vi "Drive_Globals.vi"() -> ()   [LabVIEW 2019]
uses:
  Subsystems/Drive/Drive_Cluster.ctl
  Subsystems/Drive/Drive_States.ctl
panel:
  in  "Swerve_IMU":string="Swerve_IMU"
  in  "Swerve_Drive_Front_Right_Ref":string="Swerve_Drive_Front_Right_Ref"
  in  "Swerve_Azimuth_Front_Right_Ref":string="Swerve_Azimuth_Front_Right_Ref"
  in  "Swerve_Drive_Back_Right_Ref":string="Swerve_Drive_Back_Right_Ref"
  in  "Swerve_Azimuth_Back_Right_Ref":string="Swerve_Azimuth_Back_Right_Ref"
  in  "Swerve_Drive_Back_Left_Ref":string="Swerve_Drive_Back_Left_Ref"
  in  "Swerve_Azimuth_Back_Left_Ref":string="Swerve_Azimuth_Back_Left_Ref"
  in  "Swerve_Drive_Front_Left_Ref":string="Swerve_Drive_Front_Left_Ref"
  in  "Swerve_Azimuth_Front_Left_Ref":string="Swerve_Azimuth_Front_Left_Ref"
  in  "Azimuth_Motor_Back_Right":dbl
  in  "Azimuth_Motor_Back_Left":dbl
  in  "Azimuth_Motor_Front_Left":dbl
  in  "Azimuth_Motor_Front_Right":dbl
  in  "Drive_Motor_Back_Right":dbl
  in  "Drive_Motor_Back_Left":dbl
  in  "Drive_Motor_Front_Left":dbl
  in  "Drive_Motor_Front_Right":dbl
  in  "Drive_Execute_Ref":string="Drive_Execute_Ref"
  in  "Drive_Set_Ref":string="Drive_Set_Ref"
  in  "Drive_Execute_Notifier":refnum<notifier>
  in  "Drive_Set_Notifier":refnum<notifier>
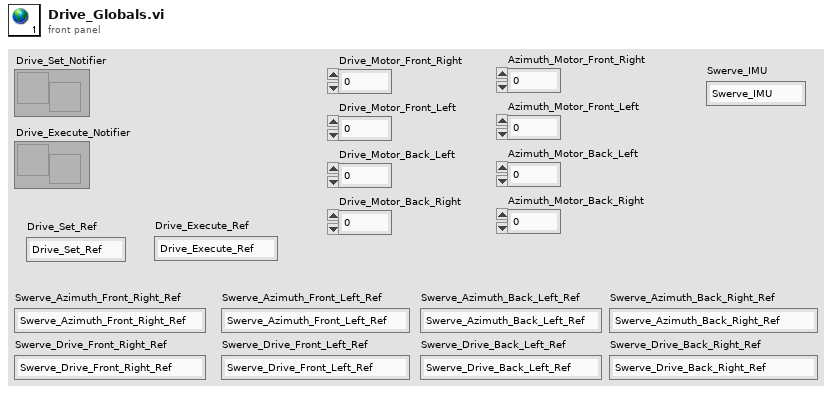
[diagram p1: front panel]
diagram:
